vi "Gen Stage 1 Update Name.vi"(6 "Channels to Create":T1[](array[typedef]), 7 "Staus":refnum<vi>, 8 "error in":errorcluster, 9 "Overlay Icon":refnum<class "Icon.lvclass">, 10 "New Subname":string, 11 "Template Project Path":path) -> (0 "error out":errorcluster)   [LabVIEW 2021, in "Plugin Generator.lvlib"]
uses:
  Plugin Generator.lvlib
  <vilib>/CIF Foundation/CIF Core/Channels/ChannelRegistrar/typedef/Channel Definition for Scripting.ctl
  <vilib>/CIF Foundation/CIF Channels Core/CIFChannels/Typedef/Direction.ctl
  <vilib>/CIF Foundation/CIF Core/Channels/ChannelRegistrar/typedef/Registered Channel Types.ctl
  <vilib>/LabVIEW Icon API/lv_icon/Classes/Icon/Icon.lvclass
  <vilib>/CIF Foundation/CIF LabVIEW Scripting/LV Scripting/LV Scripting Utilities.lvlib
  <vilib>/CIF Foundation/CIF Channels Core/CIFChannels/CIFChannels.lvclass
  <vilib>/CIF Foundation/CIF Core/Channels/ChannelRegistrar/ChannelRegistrar.lvlib
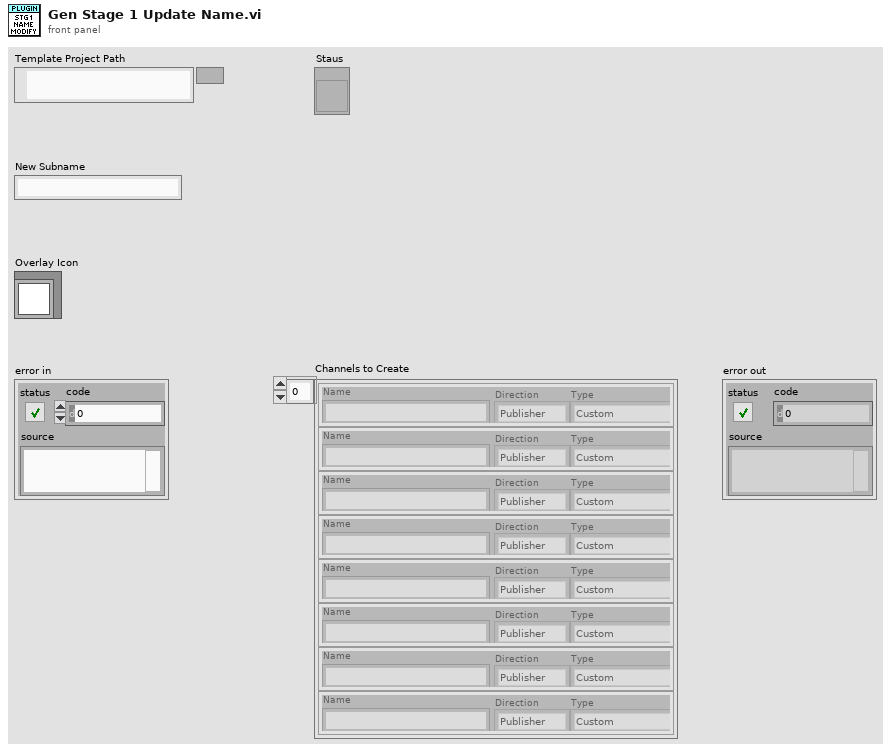
[diagram p1: front panel]
types:
  T1 = typedef "ChannelRegistrar.lvlib/Channel Definition for Scripting.ctl" = cluster{"Name":string, "Direction":T2, "Type":T3}
  T2 = typedef "CIFChannels.lvclass/Direction.ctl" = enum16{"Publisher", "Subscriber"}
  T3 = typedef "ChannelRegistrar.lvlib/Registered Channel Types.ctl" = enum16{"Custom", "Double_Tag", "I64_Tag", "U64_Tag", "U8_FIFO", "CAN_FIFO", "L2Enet_FIFO", "DAQ_FIFO", "Universal_FIFO", "String_Tag"}
  T4 = cluster{"Library Name":string, "Update Folder Name":bool}[]
  T5 = typedef "LV Scripting Utilities.lvlib/Target References.ctl" = cluster{"Target Reference":refnum<vi>, "VI References":refnum<vi>[], "Library References":refnum<vi>[], "Build References":refnum<vi>[]}
  T6 = typedef "LV Scripting Utilities.lvlib/Library Map.ctl" = map{string, refnum<vi>}
  T7 = typedef "LV Scripting Utilities.lvlib/VI Map.ctl" = map{string, refnum<vi>}
  T8 = typedef "Plugin Generator.lvlib/Proto Names.ctl" = cluster{"PascalCase":string, "snake_case":string}
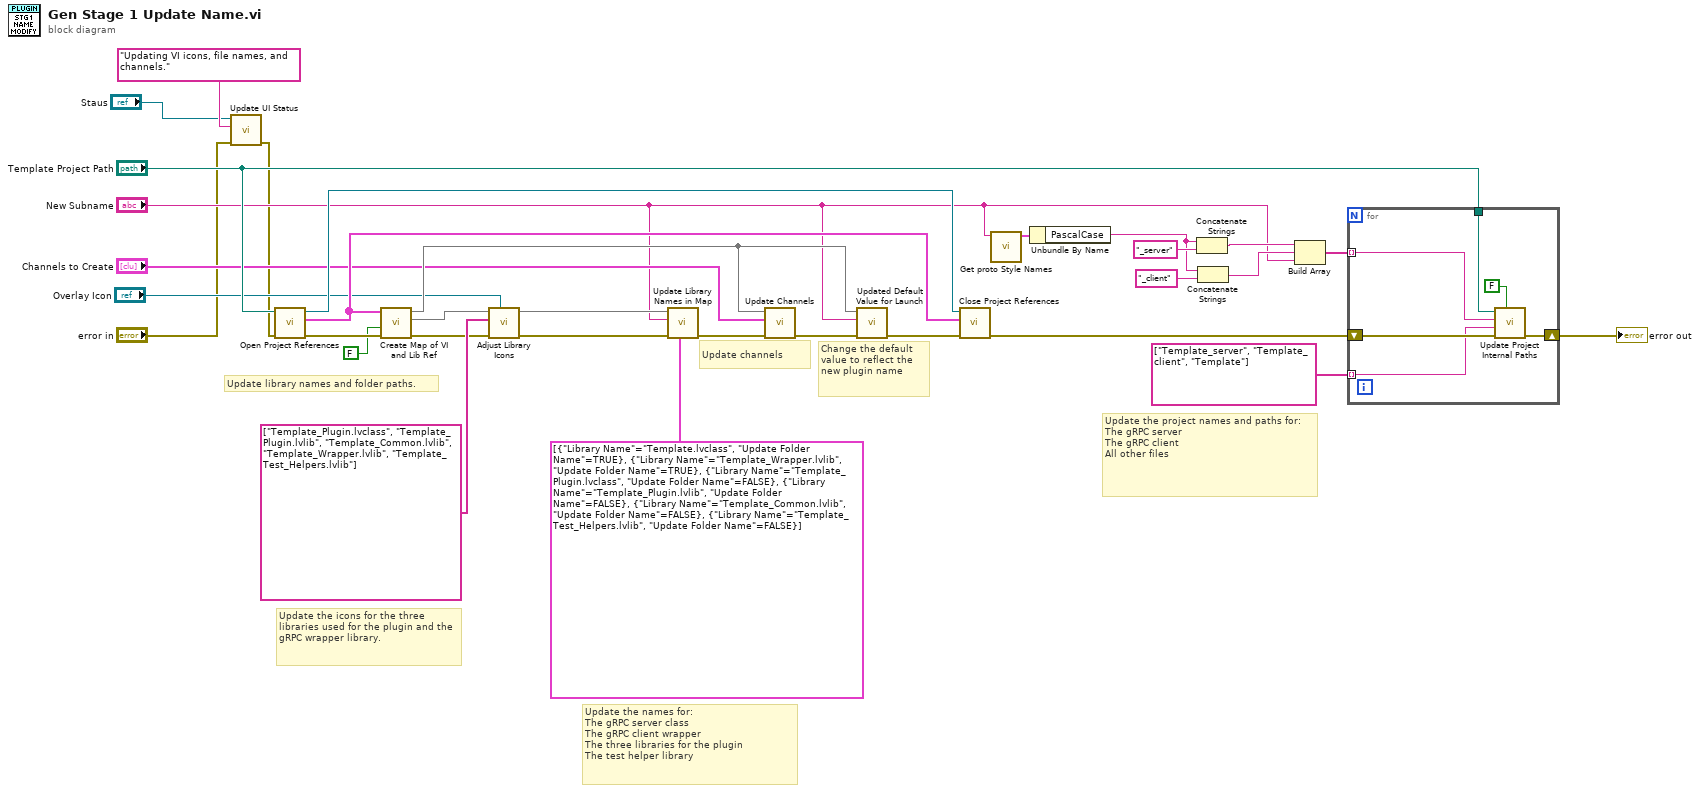
[diagram p0: block diagram]
diagram:
  # "Update the project names and paths for:\nThe gRPC server \nThe gRPC client \nAll other files"
  # "Update channels"
  # "Update library names and folder paths."
  # "Change the default value to reflect the new plugin name"
  # "Update the names for:\nThe gRPC server class\nThe gRPC client wrapper\nThe three libraries for the plugin\nThe test helper library"
  # "Update the icons for the three libraries used for the plugin and the gRPC wrapper library."
  n1 = call "Update UI Status.vi"("error in"="error in", "Status to Display"="Updating VI icons, file names, and channels." ("To display"), "String in"="Staus") -> ("error out"=w4:errorcluster)  [unwired: 8 in]
  n2 = call <vilib>:"Open Project References.vi"("error in"=w4, "Project Path"="Template Project Path") -> ("error out"=w25:errorcluster, "VI, Library, and Build References"=w22:T5[], "Project Reference"=w23:refnum<vi>)  [unwired: 7 in]
  n3 = call <vilib>:"Create Map of VI and Lib Ref.vi"("error in"=w25, "RT Target"=FALSE, "VI, Library, and Build References"=w22) -> ("error out"=w29:errorcluster, "Library Map"=w30:T6, "VI Map"=w20:T7)  [unwired: 5 in, 1 out]
  n4 = call <vilib>:"Adjust Library Icons.vi"("Overlay Icon"="Overlay Icon", "error in"=w29, "Library Names"=string[] ["Template_Plugin.lvclass", "Template_Plugin.lvlib", "Template_Common.lvlib", "Template_Wrapper.lvlib", "Template_Test_Helpers.lvlib"], "Library Map in"=w30) -> ("error out"=w1:errorcluster, "Library Map out"=w28:map{string, refnum<vi>})  [unwired: 5 in, 1 out]
  n5 = call <vilib>:"Update Library Names in Map.vi"("Libraries"=T4 [{"Library Name"="Template.lvclass", "Update Folder Name"=TRUE}, {"Library Name"="Template_Wrapper.lvlib", "Update Folder Name"=TRUE}, {"Library Name"="Template_Plugin.lvclass", "Update Folder Name"=FALSE}, {"Library Name"="Template_Plugin.lvlib", "Update Folder Name"=FALSE}, {"Library Name"="Template_Common.lvlib", "Update Folder Name"=FALSE}, {"Library Name"="Template_Test_Helpers.lvlib", "Update Folder Name"=FALSE}], "error in"=w1, "New Subname"="New Subname", "Library Map"=w28) -> ("error out"=w19:errorcluster)  [unwired: 6 in, 1 out]
  n6 = call "Update Channels.vi"("error in"=w19, "Channels to Create"="Channels to Create", "VI Map"=w20) -> ("error out"=w18:errorcluster)  [unwired: 8 in]
  n7 = call "Updated Default Value for Launch.vi"("error in"=w18, "New Subname"="New Subname", "Name to VI Map"=w20) -> ("error out"=w24:errorcluster)  [unwired: 8 in]
  n8 = call <vilib>:"Close Project References.vi"("error in"=w24, "VI, Library, and Build References"=w22, "Project Reference"=w23) -> ("error out"=w15:errorcluster)  [unwired: 8 in]
  n9 = call "Get proto Style Names.vi"("Input Name"="New Subname") -> ("Proto Names"=w14:T8)  [unwired: 10 in]
  n10 = Unbundle By Name(w14) -> ("PascalCase"=w12:string)
  n11 = Concatenate Strings(w12, "_server" ("Replace Subname")) -> (w10:string)
  n12 = Concatenate Strings(w12, "_client" ("Replace Subname")) -> (w9:string)
  n13 = Build Array(w10, w9, "New Subname") -> (w8:string[])
  n14 = for {
    tunnel: "Template Project Path" -> [w37]
    shift-right: [w38] -> w32
    shift-left: w15 -> [w35]
    tunnel: w8 -> [w33] mode=indexing
    tunnel: string[] ["Template_server", "Template_client", "Template"] -> [w34] mode=indexing
    n15 = call <vilib>:"Update Project Internal Paths.vi"("Rename Project"=FALSE, "error in (no error)"=w35, "Replace Subname"=w34, "New Subname"=w33, "Project Path"=w37) -> ("error out"=w38:errorcluster)  [unwired: 6 in]
  }
  "error out" <- w32
